vi "Friction (DBL).vi"(2 "offset":dbl format="%.2f", 3 "gain":dbl format="%.2f", 4 "input point":dbl format="%.2f") -> (1 "output point":dbl format="%.2f")   [LabVIEW 2020, in "NI_AdvCtrl_nonlinear.lvlib"]
doc: "LabVIEW no longer supports this VI. You can obtain similar functionality by installing the LabVIEW Simulation Module.\n\nRealizes a discontinuity at zero but guarantees the linear behavior elsewhere."
uses:
  <vilib>/addons/control/advanced/NI_AdvCtrl_nonlinear.lvlib
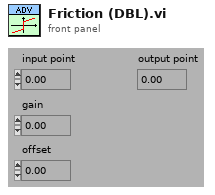
[diagram p1: front panel]
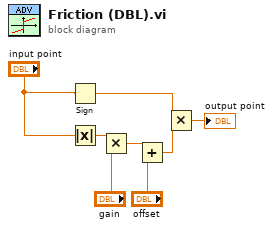
[diagram p0: block diagram]
diagram:
  n1 = Sign(1:"input point") -> (0:w6:dbl)
  n2 = Absolute Value(x="input point") -> (abs(x)=w3:dbl)
  n3 = Multiply(x=w3, y="gain") -> (x*y=w4:dbl)
  n4 = Add(x=w4, y="offset") -> (x+y=w7:dbl)
  n5 = Multiply(x=w6, y=w7) -> (x*y=→"output point":dbl)
